vi "NicmosOpenSynchronization.vi"(9 "error out":errorcluster caption="error in (no error)") -> (2 "Synchronization":T1, 6 "error in (no error)":errorcluster caption="error out")   [LabVIEW 2009]
uses:
  Controls/NicmosSynchronization.ctl
  Controls/NICMOS.COMMAND.QUEUE.ctl
  Controls/NICMOS.COMMAND.ctl
  Controls/NICMOS.COMMANDBASIC.ctl
  Controls/NICMOS.READOUT.ctl
  Controls/NICMOS.FILTERCOMMAND.ctl
  Controls/NICMOS.FILTER.ctl
  Controls/NICMOS.STATE.NOTIFIER.ctl
  Controls/NICMOS.STATE.ctl
  Controls/NICMOS.DATA.NOTIFIER.ctl
  Controls/NICMOS.DATA.ctl
  Controls/NICMOS.DATA.QUEUE.ctl
  Controls/NICMOS.RAW.NOTIFIER.ctl
  Controls/NICMOS.RAW.ctl
  Controls/NICMOS.TEMPERATURE.NOTIFIER.ctl
  Controls/NICMOS.TEMPERATURE.ctl
  Controls/NICMOS.READOUT.NOTIFIER.ctl
  Controls/NICMOS.FILTER.NOTIFIER.ctl
  Controls/NICMOS.MASKBANKS.NOTIFIER.ctl
  Controls/NICMOS.MASKBANKS.ctl
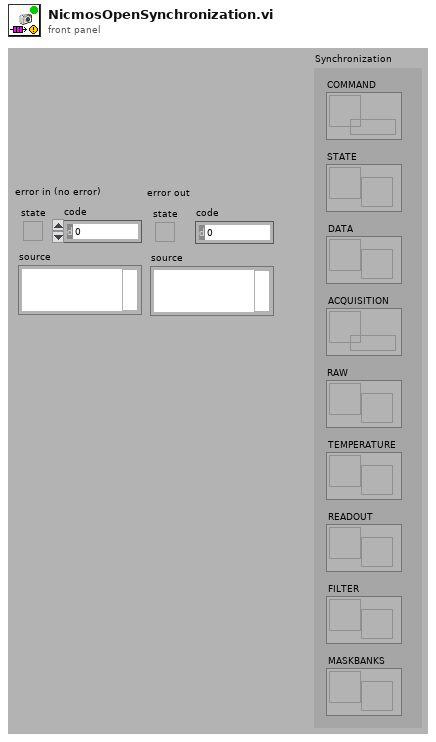
[diagram p1: front panel]
types:
  T1 = typedef "NicmosSynchronization.ctl" = cluster{"COMMAND":T2, "STATE":T3, "DATA":T4, "ACQUISITION":T5, "RAW":T6, "TEMPERATURE":T7, "READOUT":T8, "FILTER":T9, "MASKBANKS":T10}
  T2 = typedef "NICMOS.COMMAND.QUEUE.ctl" = refnum<queue>
  T3 = typedef "NICMOS.STATE.NOTIFIER.ctl" = refnum<notifier>
  T4 = typedef "NICMOS.DATA.NOTIFIER.ctl" = refnum<notifier>
  T5 = typedef "NICMOS.DATA.QUEUE.ctl" = refnum<queue>
  T6 = typedef "NICMOS.RAW.NOTIFIER.ctl" = refnum<notifier>
  T7 = typedef "NICMOS.TEMPERATURE.NOTIFIER.ctl" = refnum<notifier>
  T8 = typedef "NICMOS.READOUT.NOTIFIER.ctl" = refnum<notifier>
  T9 = typedef "NICMOS.FILTER.NOTIFIER.ctl" = refnum<notifier>
  T10 = typedef "NICMOS.MASKBANKS.NOTIFIER.ctl" = refnum<notifier>
  T11 = typedef "NICMOS.MASKBANKS.ctl" = cluster{"MaskList":cluster{"X":i32, "Y":i32, "NX":i32, "NY":i32}[], "Reform X":i32, "Reform Y":i32}[]
  T12 = typedef "NICMOS.FILTER.ctl" = string
  T13 = typedef "NICMOS.READOUT.ctl" = cluster{"Readout":i32, "Deglitch":i32, "Framerate":dbl[unit], "Bank":i32}
  T14 = typedef "NICMOS.TEMPERATURE.ctl" = cluster{"T1":dbl, "T2":dbl}
  T15 = typedef "NICMOS.DATA.ctl" = cluster{"DATA":i32[][][], "INDEX":i32}
  T16 = typedef "NICMOS.COMMAND.ctl" = cluster{"Command":T17, "READOUT":T13, "FILTERCOMMAND":T18, "ACQUISITION":i32, "Done":refnum<k4>}
  T17 = typedef "NICMOS.COMMANDBASIC.ctl" = enum16{"WRITE BANKS", "SET FILTER", "HOME FILTER", "QUERY TEMP", "CONFIGURE", "START", "ACQUISITION", "STOP", "QUIT"}
  T18 = typedef "NICMOS.FILTERCOMMAND.ctl" = cluster{"FILTER":T12, "INIT":bool}
  T19 = typedef "NICMOS.STATE.ctl" = enum16{"IDLE", "WRITING BANKS", "SETTING FILTER", "HOMING FILTER", "QUERYING TEMP", "CONFIGURING", "STARTING", "RUNNING", "HALTING", "STOPPED"}
  T20 = typedef "NICMOS.RAW.ctl" = u16[][][]
  T21 = cluster{"queue out":refnum<queue>, "notifier out":refnum<notifier>, "notifier out":refnum<notifier>, "queue out":refnum<queue>, "notifier out":refnum<notifier>, "notifier out":refnum<notifier>, "notifier out":refnum<notifier>, "notifier out":refnum<notifier>, "notifier out":refnum<notifier>}
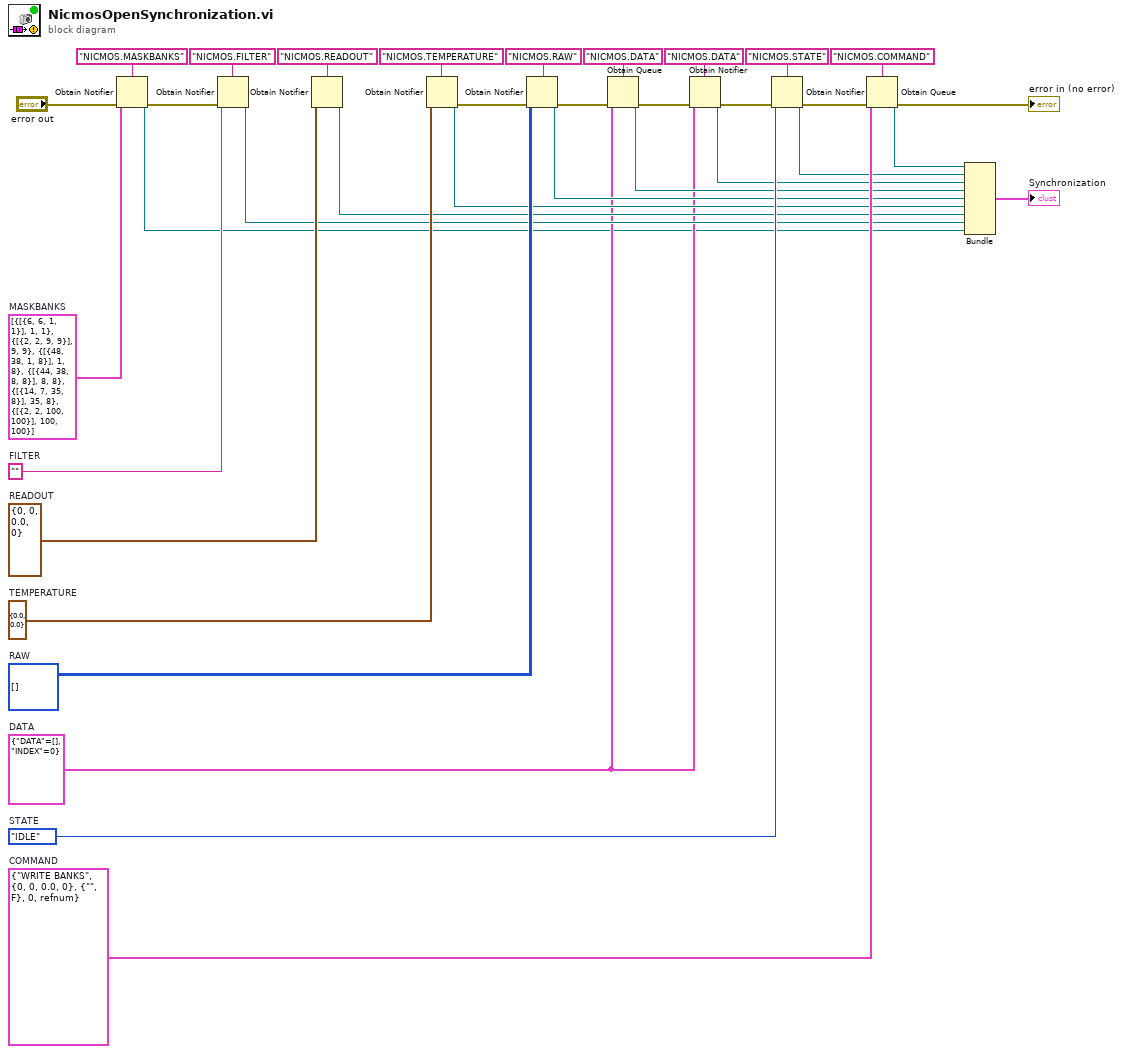
[diagram p0: block diagram]
diagram:
  w2 = T11 [{"MaskList"=[{"X"=6, "Y"=6, "NX"=1, "NY"=1}], "Reform X"=1, "Reform Y"=1}, {"MaskList"=[{"X"=2, "Y"=2, "NX"=9, "NY"=9}], "Reform X"=9, "Reform Y"=9}, {"MaskList"=[{"X"=48, "Y"=38, "NX"=1, "NY"=8}], "Reform X"=1, "Reform Y"=8}, {"MaskList"=[{"X"=44, "Y"=38, "NX"=8, "NY"=8}], "Reform X"=8, "Reform Y"=8}, {"MaskList"=[{"X"=14, "Y"=7, "NX"=35, "NY"=8}], "Reform X"=35, "Reform Y"=8}, {"MaskList"=[{"X"=2, "Y"=2, "NX"=100, "NY"=100}], "Reform X"=100, "Reform Y"=100}]  # MASKBANKS
  w12 = T12 ""  # FILTER
  w15 = T13 {"Readout"=0, "Deglitch"=0, "Framerate"=0.0, "Bank"=0}  # READOUT
  w18 = T14 {"T1"=0.0, "T2"=0.0}  # TEMPERATURE
  w6 = T15 {"DATA"=[], "INDEX"=0}  # DATA
  w26 = T16 {"Command"=enum."WRITE BANKS", "READOUT"={"Readout"=0, "Deglitch"=0, "Framerate"=0.0, "Bank"=0}, "FILTERCOMMAND"={"FILTER"="", "INIT"=FALSE}, "ACQUISITION"=0, "Done"=refnum}  # COMMAND
  w28 = NICMOS.STATE."IDLE"  # STATE
  w27 = T20 []  # RAW
  n1 = Obtain Notifier(name (unnamed)="NICMOS.MASKBANKS" ("nom (aucun)"), notification data type=w2, error in (no error)="error out") -> (notifier out=w1:refnum<notifier>, error out=w3:errorcluster)  [unwired: 1 in, 1 out]
  n2 = Obtain Notifier(name (unnamed)="NICMOS.FILTER" ("nom (aucun)"), notification data type=w12, error in (no error)=w3) -> (notifier out=w11:refnum<notifier>)  [unwired: 1 in, 2 out]
  n3 = Obtain Notifier(name (unnamed)="NICMOS.READOUT" ("nom (aucun)"), notification data type=w15) -> (notifier out=w14:refnum<notifier>)  [unwired: 2 in, 2 out]
  n4 = Obtain Notifier(name (unnamed)="NICMOS.TEMPERATURE" ("nom (aucun)"), notification data type=w18) -> (notifier out=w17:refnum<notifier>, error out=w19:errorcluster)  [unwired: 2 in, 1 out]
  n5 = Obtain Notifier(name (unnamed)="NICMOS.RAW" ("nom (aucun)"), notification data type=w27, error in (no error)=w19) -> (notifier out=w21:refnum<notifier>, error out=w29:errorcluster)  [unwired: 1 in, 1 out]
  n6 = Obtain Queue(name (unnamed)="NICMOS.DATA" ("nom (aucun)"), element data type=w6, error in (no error)=w29) -> (queue out=w22:refnum<queue>, error out=w10:errorcluster)  [unwired: 2 in, 1 out]
  n7 = Obtain Notifier(name (unnamed)="NICMOS.DATA" ("nom (aucun)"), notification data type=w6, error in (no error)=w10) -> (notifier out=w7:refnum<notifier>, error out=w9:errorcluster)  [unwired: 1 in, 1 out]
  n8 = Obtain Notifier(name (unnamed)="NICMOS.STATE" ("nom (aucun)"), notification data type=w28, error in (no error)=w9) -> (notifier out=w23:refnum<notifier>, error out=w31:errorcluster)  [unwired: 1 in, 1 out]
  n9 = Obtain Queue(name (unnamed)="NICMOS.COMMAND" ("nom (aucun)"), element data type=w26, error in (no error)=w31) -> (queue out=w24:refnum<queue>, error out=→"error in (no error)":errorcluster)  [unwired: 2 in, 1 out]
  n10 = Bundle("queue out"=w24, "notifier out"=w23, "notifier out"=w7, "queue out"=w22, "notifier out"=w21, "notifier out"=w17, "notifier out"=w14, "notifier out"=w11, "notifier out"=w1) -> (→"Synchronization":T21)  [unwired: 1 in]
